vi "Validate Inputs.vi"(11 "Network Session Handler in":refnum<class "Network Session Handler.lvclass">) -> (0 "error out":errorcluster)   [LabVIEW 2017, in "Network Interface.lvlib" / "Network Session Handler.lvclass"]
uses:
  <vilib>/gpm_packages/@cs/Network-sink/Source/Network Interface/Network Session Handler/Network Session Handler.lvclass
  <vilib>/gpm_packages/@cs/Network-sink/Source/Network Interface/IMessagingProtocol/IMessagingProtocol.lvclass
  <vilib>/gpm_packages/@cs/Network-sink/Source/Network Interface/IConnectionFactory/IConnectionFactory.lvclass
  <vilib>/gpm_packages/@cs/Network-sink/Source/Network Interface/Network Session Handler/Network Session Handler.lvclass/Network Session Handler.ctl
  <vilib>/ErrorRing/Error Ring.xnode
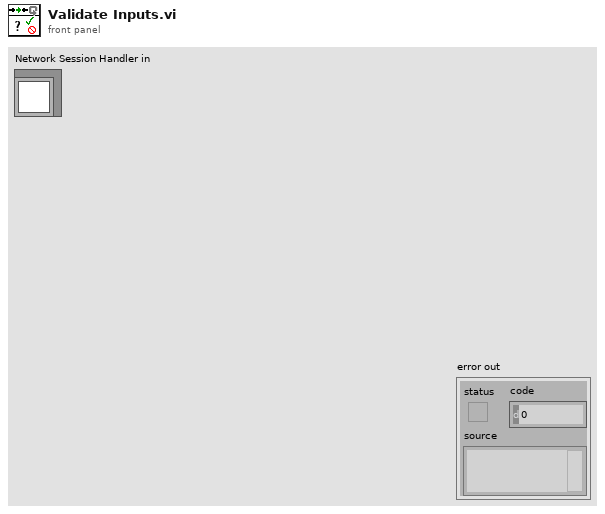
[diagram p1: front panel]
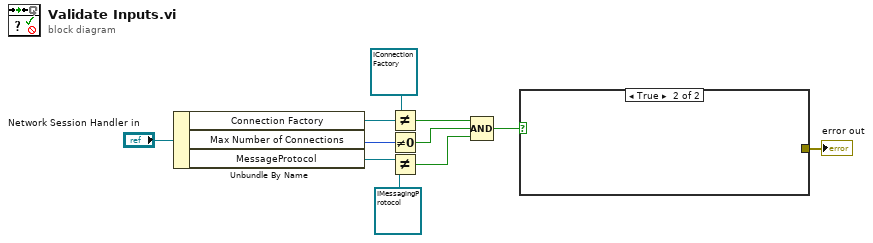
[diagram p0: block diagram]
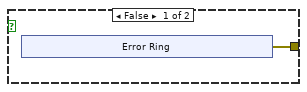
[diagram p2: hidden frame]
diagram:
  n1 = Unbundle By Name("Network Session Handler in") -> ("Connection Factory"=w7:refnum<class "IConnectionFactory.lvclass">, "Max Number of Connections"=w10:i32, "MessageProtocol"=w8:refnum<class "IMessagingProtocol.lvclass">)
  n2 = Not Equal?(x=refnum<class "IConnectionFactory.lvclass"> refnum, y=w7) -> (x != y?=w5:bool)
  n3 = Not Equal To 0?(x=w10) -> (x != 0?=w4:bool)
  n4 = Not Equal?(x=w8, y=refnum<class "IMessagingProtocol.lvclass"> refnum ("x")) -> (x != y?=w3:bool)
  n5 = Compound Arithmetic op=AND(w5, w4, w3) -> (w2:bool)
  n6 = case shown="True" w2 {
    tunnel: [w12 _] -> w1
    frame False {
      n7 = xnode "Error Ring"() -> ("error out"=w12:errorcluster)
    }
    frame True {
    }
  }
  "error out" <- w1
